vi "Render.vi"(7 "Renderer":refnum<class "Renderer.lvclass">, 8 "error in (no error)":errorcluster, 10 "Camera":refnum<class "Camera.lvclass">, 11 "Asteroid in":refnum<class "Asteroid.lvclass">) -> (0 "error out":errorcluster)   [LabVIEW 2021, in "Asteroid.lvclass"]
uses:
  Asteroid.lvclass
  Camera/Camera.lvclass
  Renderer/Renderer.lvclass
  Asteroid.lvclass/Asteroid.ctl
  Re-use Libraries/Vector 2D/Vector 2D.lvclass
  Resource Manager/Resource Manager.lvclass
  Element/Element.lvclass
  LabSDL2/Source/Libraries/LibSDL2 Wrapper/LibSDL2.lvlib
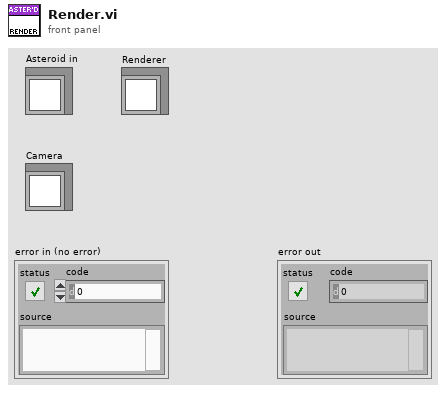
[diagram p1: front panel]
types:
  T1 = typedef "LibSDL2.lvlib/Rectangle.ctl" = cluster{"x":i32, "y":i32, "Width":i32, "Height":i32}
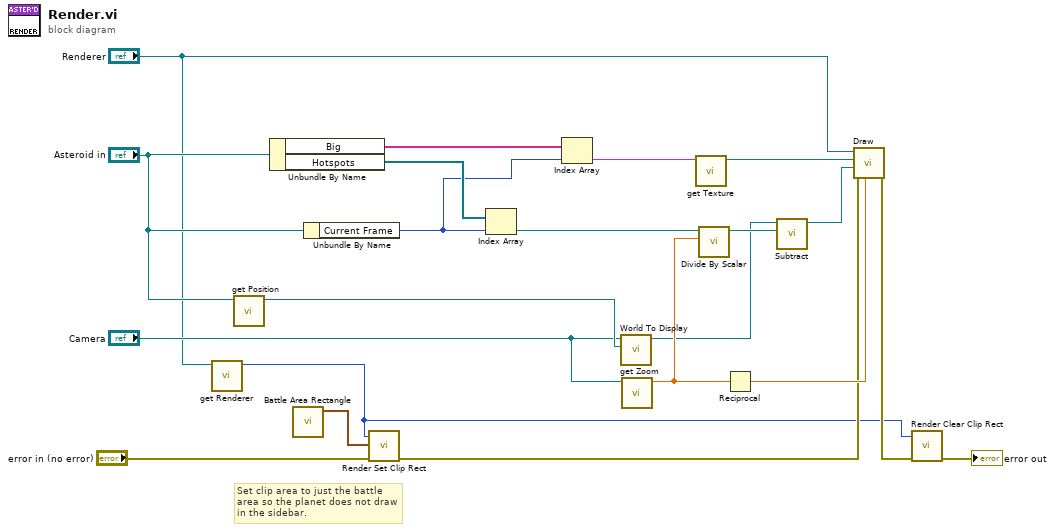
[diagram p0: block diagram]
diagram:
  # "Set clip area to just the battle area so the planet does not draw in the sidebar."
  n1 = call-dynamic "get Renderer.vi"("Renderer in"="Renderer") -> ("Renderer"=w1:u32)  [unwired: 10 in]
  n2 = call "get Position.vi"("Element in"="Asteroid in") -> ("Position"=w16:refnum<class "Vector 2D.lvclass">)  [unwired: 10 in]
  n3 = Unbundle By Name("Asteroid in") -> ("Big"=w21:string[], "Hotspots"=w19:refnum<class "Vector 2D.lvclass">[])
  n4 = call "Battle Area Rectangle.vi"() -> ("Viewport"=w3:T1)  [unwired: 11 in]
  n5 = Unbundle By Name("Asteroid in") -> ("Current Frame"=w17:i32)
  n6 = call "Render Set Clip Rect.vi"("error in"="error in (no error)", "Rectangle"=w3, "Renderer Pointer"=w1) -> ("error out"=w4:errorcluster)  [unwired: 7 in, 1 out]
  n7 = Index Array(array=w19, index=w17) -> (element=w9:refnum<class "Vector 2D.lvclass">)
  n8 = Index Array(array=w21, index=w17) -> (element=w20:string)
  n9 = call "World To Display.vi"("World Position"=w16, "Camera in"="Camera") -> ("Display Position"=w8:refnum<class "Vector 2D.lvclass">)  [unwired: 9 in]
  n10 = call "get Zoom.vi"("Camera in"="Camera") -> ("Zoom Level"=w12:sgl)  [unwired: 10 in]
  n11 = call "get Texture.vi"("Texture Name"=w20) -> ("Texture"=w15:refnum<class "Texture.lvclass">)  [unwired: 10 in]
  n12 = call "Divide By Scalar.vi"("x"=w12, "A"=w9) -> ("Ax"=w11:refnum<class "Vector 2D.lvclass">)  [unwired: 9 in]
  n13 = Reciprocal(x=w12) -> (1/x=w14:sgl)
  n14 = call "Subtract.vi"("B"=w11, "A"=w8) -> ("A-B"=w10:refnum<class "Vector 2D.lvclass">)  [unwired: 9 in]
  n15 = call "Draw.vi"("Scale"=w14, "error in (no error)"=w4, "Destination"=w10, "Texture"=w15, "Renderer"="Renderer") -> ("error out"=w7:errorcluster)  [unwired: 6 in]
  n16 = call "Render Clear Clip Rect.vi"("error in"=w7, "Renderer Pointer"=w1) -> ("error out"=→"error out":errorcluster)  [unwired: 8 in, 1 out]
